vi "XIPIN_Constant_1_1.vi"   [LabVIEW 2017]
doc: "Gives a constant signed value.\n------------------------------------\n<b>Need License</b> : No"
uses:
  <vilib>/rvi/XilinxIP/XIPIN_XNode/niFpgaXIPIN.xnode
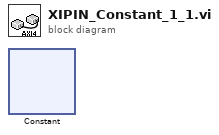
[diagram p0: block diagram]
diagram:
  n1 = xnode ("Constant")() -> ()
